vi "Get PS Status.vi"(8 "error in (no error)":errorcluster, 11 "PS Control Actor in":refnum<class "PS Control Actor.lvclass">) -> (0 "error out":errorcluster, 3 "PS Control Actor out":refnum<class "PS Control Actor.lvclass">)   [LabVIEW 2019, in "PS Control Actor.lvlib" / "PS Control Actor.lvclass"]
uses:
  PS Control Actor.lvclass
  <vilib>/ActorFramework/Actor/Actor.lvclass
  PS Control Actor Messages/Get PS Status Msg/Get PS Status Msg.lvclass
  PS Driver/PS Driver.lvclass
  Applications/National Instruments/LabVIEW 2019 64-bit/vi.lib/ActorFramework/Actor/Actor.lvclass
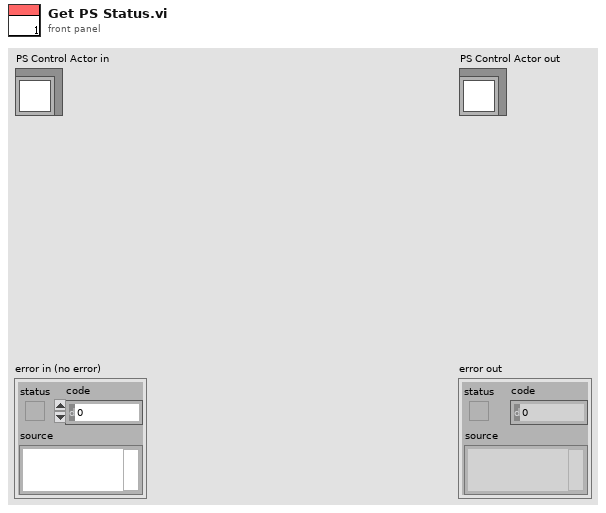
[diagram p1: front panel]
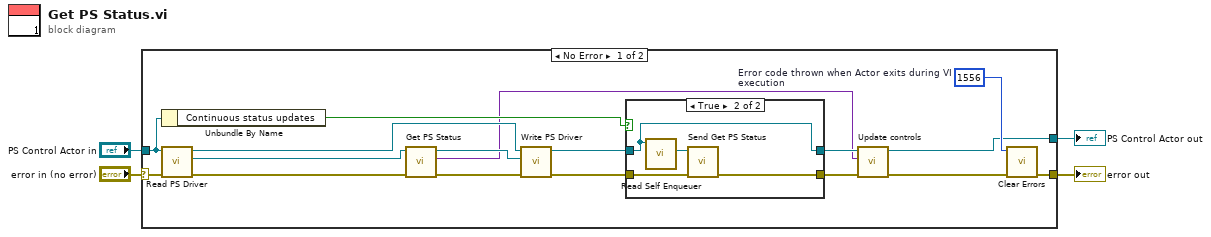
[diagram p0: block diagram]
diagram:
  n1 = case shown="No Error" "error in (no error)" {
    selector: "error in (no error)" -> [w10 w29]
    tunnel: [w20 w29] -> w3
    tunnel: [w6 w28] -> w1
    tunnel: "PS Control Actor in" -> [w18 w28]
    frame No Error {
      w21 = 1556  # Error code thrown when Actor exits during VI execution
      n2 = Unbundle By Name(w18) -> ("Continuous status updates"=w19:bool)
      n3 = call-dynamic "Read PS Driver.vi"("error in (no error)"=w10, "PS Control Actor in"=w18) -> ("error out"=w13:errorcluster, "PS Driver.lvlib:PS Driver.lvclass"=w12:refnum<class "PS Driver.lvclass">, "PS Control Actor out"=w17:refnum<class "PS Control Actor.lvclass">)  [unwired: 7 in]
      n4 = call-dynamic "Get PS Status.vi"("error in (no error)"=w13, "PS Driver.lvlib:PS Driver.lvclass"=w12) -> ("error out"=w14:errorcluster, "Status out"=w7:variant, "PS Driver.lvlib:PS Driver.lvclass out"=w11:refnum<class "PS Driver.lvclass">)  [unwired: 7 in]
      n5 = call-dynamic "Write PS Driver.vi"("error in (no error)"=w14, "PS Driver.lvlib:PS Driver.lvclass"=w11, "PS Control Actor in"=w17) -> ("error out"=w15:errorcluster, "PS Control Actor out"=w16:refnum<class "PS Control Actor.lvclass">)  [unwired: 7 in]
      n6 = case shown="True" w19 {
        tunnel: w16 -> [w22 w24]
        tunnel: w15 -> [w23 w26]
        tunnel: [w23 w25] -> w8
        tunnel: [w22 w24] -> w9
        frame False {
        }
        frame True {
          n7 = call <vilib>:"Read Self Enqueuer.vi"("Actor"=w24) -> ("Self Enqueuer"=w27:refnum<class "Message Enqueuer.lvclass">)  [unwired: 10 in]
          n8 = call "Send Get PS Status.vi"("error in (no error)"=w26, "Message Enqueuer"=w27) -> ("error out"=w25:errorcluster)  [unwired: 8 in, 1 out]
        }
      }
      n9 = call "Update controls.vi"("error in (no error)"=w8, "New control values"=w7, "PS Control Actor in"=w9) -> ("error out"=w5:errorcluster, "PS Control Actor out"=w6:refnum<class "PS Control Actor.lvclass">)  [unwired: 7 in]
      n10 = call <vilib>:"Clear Errors.vi"("error in (no error)"=w5, "specific error code to clear (0: all)"=w21) -> ("error out"=w20:errorcluster)  [unwired: 4 in, 1 out]
    }
    frame Error {
    }
  }
  "error out" <- w3
  "PS Control Actor out" <- w1
